vi "Configure Hardware.vi"(8 "error in (no error)":errorcluster, 11 "Hardware Resources in":T1={"DAQmx Task"="", "Counter(s)"="Dev2/ctr0", "samples per readout"=0}) -> (0 "error out":errorcluster, 3 "Hardware Resources out":T1={"DAQmx Task"="", "Counter(s)"="Dev2/ctr0", "samples per readout"=0})   [LabVIEW 2013, in "Acquisition.lvlib"]
doc: "Configure the hardware."
uses:
  Acquisition.lvlib
  Counter Configuration.ctl
  <vilib>/DAQmx/create/channels.llb/DAQmx Create Channel (CI-Period).vi
  <vilib>/DAQmx/configure/timing.llb/DAQmx Timing (Implicit).vi
  <resource>/objmgr/daqmx.rc
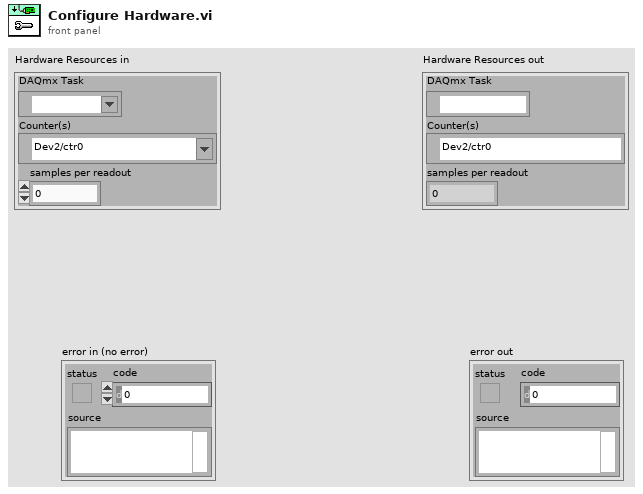
[diagram p1: front panel]
types:
  T1 = typedef "Acquisition.lvlib/Counter Configuration.ctl" = cluster{"DAQmx Task":refnum<k21>, "Counter(s)":tag, "samples per readout":i32}
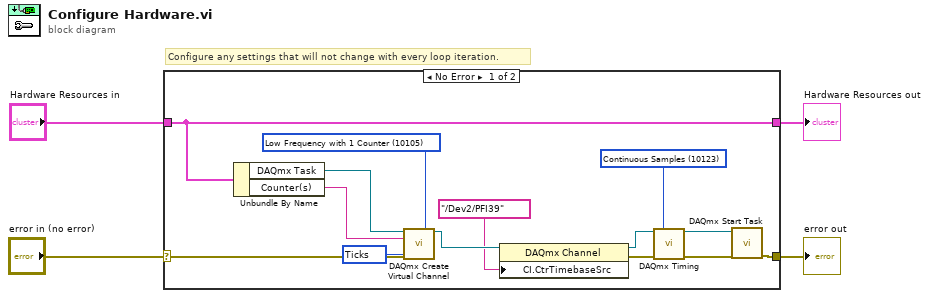
[diagram p0: block diagram]
diagram:
  # "Configure any settings that will not change with every loop iteration."
  n1 = case shown="No Error" "error in (no error)" {
    selector: "error in (no error)" -> [w16 w19]
    tunnel: [w11 w19] -> w3
    tunnel: "Hardware Resources in" -> [w15 w20]
    tunnel: [w15 w20] -> w1
    frame No Error {
      w9 = 10105 items=["Low Frequency with 1 Counter"=10105, "High Frequency with 2 Counters"=10157, "Large Range with 2 Counters"=10205] ("measurement method")
      w10 = 10304 items=["Seconds"=10364, "Ticks"=10304, "From Custom Scale"=10065] ("units")
      w14 = 10123 items=["Finite Samples"=10178, "Continuous Samples"=10123, "Hardware Timed Single Point"=12522] ("sample mode")
      n2 = Unbundle By Name(w15) -> ("DAQmx Task"=w18:refnum<k21>, "Counter(s)"=w17:tag)
      n3 = call-poly <vilib>:"DAQmx Create Virtual Channel.vi"("task in"=w18, "measurement method"=w9, "counter"=w17, "units"=w10, "error in"=w16) -> ("task out"=w8:refnum<k21>)  [unwired: 9 in, 1 out]
      n4 = property class="DAQmx Channel"(reference=w8, "CI.CtrTimebaseSrc"=tag "/Dev2/PFI39" ("Counter Source")) -> (reference out=w7:refnum<k21>, error out=w6:errorcluster)  [unwired: 1 in]
      n5 = call-poly <vilib>:"DAQmx Timing.vi"("task/channels in"=w7, "sample mode"=w14, "error in"=w6) -> ("task out"=w12:refnum<k21>, "error out"=w13:errorcluster)  [unwired: 11 in]
      n6 = call <vilib>:"DAQmx Start Task.vi"("task/channels in"=w12, "error in"=w13) -> ("error out"=w11:errorcluster)  [unwired: 12 in, 1 out]
    }
    frame Error {
    }
  }
  "Hardware Resources out" <- w1
  "error out" <- w3
